vi "mxwScript_API_XMLTemplateName_AddWizardLock.vi"(7 "wizard lock callback":path, 8 "error in (no error)":errorcluster, 9 "create new?":bool, 10 "name":string, 11 "absolutePath":string) -> (0 "error out":errorcluster, 3 "encoded absolutePath":string)   [LabVIEW 2017]
doc: "Create encoded \"absolutePath\" for adding options to the template scripting such as wizard locking."
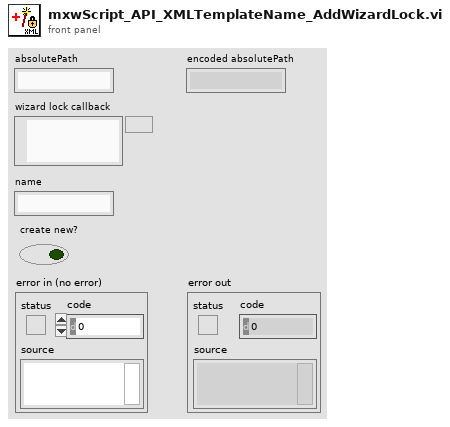
[diagram p1: front panel]
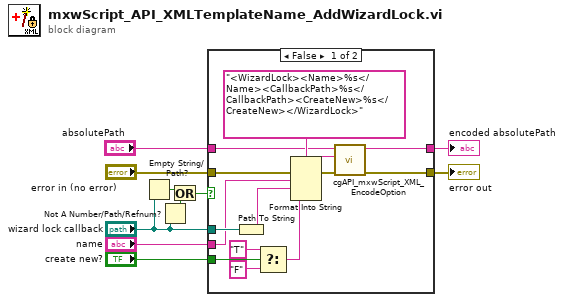
[diagram p0: block diagram]
diagram:
  n1 = Empty String/Path?(string/path="wizard lock callback") -> (empty?=w6:bool)
  n2 = Not A Number/Path/Refnum?(number/path/refnum="wizard lock callback") -> (NaN/Path/Refnum?=w5:bool)
  n3 = Or(x=w6, y=w5) -> (x .or. y?=w4:bool)
  n4 = case shown="False" w4 {
    tunnel: [w24 w26] -> w10
    tunnel: [w11 w25] -> w9
    tunnel: "error in (no error)" -> [w23 w26]
    tunnel: "absolutePath" -> [w19 w25]
    tunnel: "wizard lock callback" -> [w18 _]
    tunnel: "name" -> [w16 _]
    tunnel: "create new?" -> [w15 _]
    frame False {
      n5 = Path To String(path=w18) -> (string=w17:string)
      n6 = Select(t="T", s=w15, f="F") -> (s? t:f=w12:string)
      n7 = Format Into String(format string="<WizardLock><Name>%s</Name><CallbackPath>%s</CallbackPath><CreateNew>%s</CreateNew></WizardLock>" ("control name"), error in=w23, w16, w17, w12) -> (resulting string=w20:string, error out=w22:errorcluster)  [unwired: 1 in]
      n8 = call "cgAPI_mxwScript_XML_EncodeOption.vi"("error in (no error)"=w22, "otherXML"=w20, "normalTextString"=w19) -> ("error out"=w24:errorcluster, "encodedString"=w11:string)  [unwired: 7 out]
    }
    frame True {
    }
  }
  "error out" <- w10
  "encoded absolutePath" <- w9
